vi "Principal.vi"() -> ()   [LabVIEW 2019, in "Class 2.lvclass"]
uses:
  Class 2.lvclass
panel:
  out "ENTRADAS.BIMANUAL 1":bool
  out "Numeric":i32
  in  "stop":bool
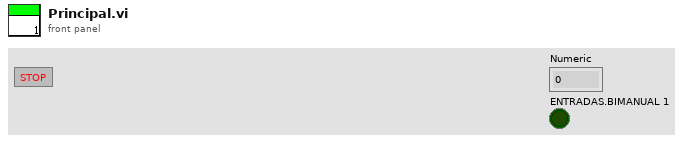
[diagram p1: front panel]
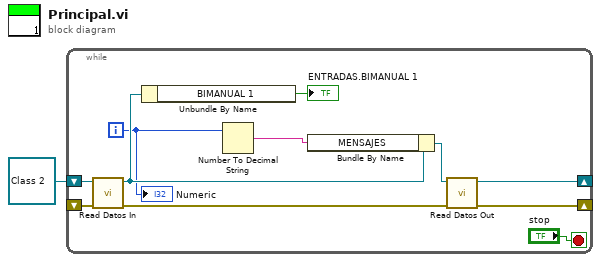
[diagram p0: block diagram]
diagram:
  n1 = while {
    shift-right: [w10] -> _
    shift-left: refnum<class "Class 2.lvclass"> refnum ("Class 2.lvclass") -> [w11]
    shift-right: [w7] -> _
    shift-left: _ -> [w9]
    i -> [w4]
    stop <- "stop" stop-if-true
    n2 = call "Read Datos In.vi"("error in (no error)"=w9, "Class 2 in"=w11) -> ("error out"=w8:errorcluster, "Class 2 out"=w5:refnum<class "Class 2.lvclass">)  [unwired: 8 in]
    n3 = Unbundle By Name(w5) -> ("BIMANUAL 1"=→"ENTRADAS.BIMANUAL 1":bool)
    n4 = Number To Decimal String(number=w4) -> (decimal integer string=w3:string)  [unwired: 1 in]
    n5 = Bundle By Name(cluster=w5, "MENSAJES"=w3) -> (w6:refnum<class "Class 2.lvclass">)
    n6 = call "Read Datos Out.vi"("error in (no error)"=w8, "Class 2 in"=w6) -> ("error out"=w7:errorcluster, "Class 2 out"=w10:refnum<class "Class 2.lvclass">)  [unwired: 8 in]
    "Numeric" <- w4
  }
